vi "Receive.vi"(8 "error in (no error)":errorcluster, 10 "Transfer Group in":refnum<class "Transfer Group.lvclass">, 11 "PXImc Transceiver in":refnum<class "PXImc Transceiver.lvclass">) -> (0 "error out":errorcluster, 2 "Transfer Group out":refnum<class "Transfer Group.lvclass">, 3 "PXImc Transceiver out":refnum<class "PXImc Transceiver.lvclass">)   [LabVIEW 2017, in "PXImc.lvlib" / "PXImc Transceiver.lvclass"]
uses:
  PXImc Transceiver.lvclass
  Builds/Data Sharing Framework/Current/Core/DSF Core.lvlibp/Classes/Transfer Group/Transfer Group.lvclass
  PXImc Transceiver.lvclass/PXImc Transceiver.ctl
  <vilib>/pximc/Acquire Read Region (U8).vi
  <vilib>/pximc/nipximc.lvlib
  Builds/Data Sharing Framework/Current/Core/DSF Core.lvlibp/Classes/Buffer/Buffer.lvclass
  Builds/Data Sharing Framework/Current/Core/DSF Core.lvlibp/Classes/Transfer/Transfer.lvclass
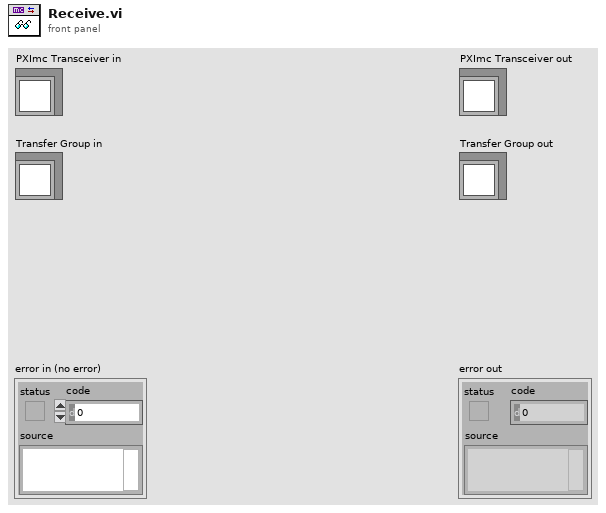
[diagram p1: front panel]
types:
  T1 = typedef "PXImc.lvlib/PXImc Transceiver.lvclass/PXImc Group Data.ctl" = cluster{"direction":T2, "transfers":T3[]}
  T2 = typedef "DSF Core.lvlibp/DSF Direction.ctl" = enum8{"Tx", "Rx"}
  T3 = typedef "PXImc.lvlib/PXImc Transceiver.lvclass/PXImc Transfer Data.ctl" = cluster{"stream id":u16, "session":refnum<k21>, "buffer size":u64}
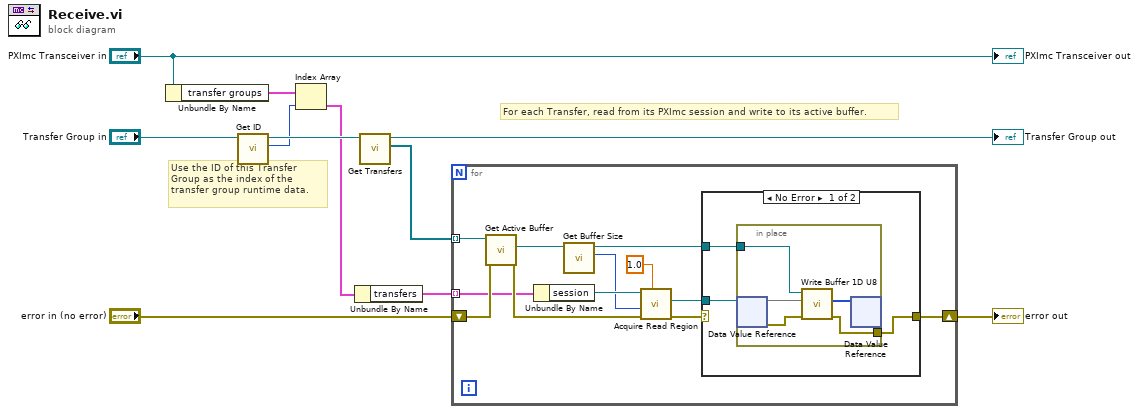
[diagram p0: block diagram]
diagram:
  # "For each Transfer, read from its PXImc session and write to its active buffer."
  # "Use the ID of this Transfer Group as the index of the transfer group runtime data."
  n1 = Unbundle By Name("PXImc Transceiver in") -> ("transfer groups"=w9:T1[])
  n2 = call "Get ID.vi"("Transfer Group in"="Transfer Group in") -> ("id"=w4:i32, "Transfer Group out"=w7:refnum<class "Transfer Group.lvclass">)  [unwired: 9 in]
  n3 = Index Array(array=w9, index=w4) -> (element=w3:T1)
  n4 = Unbundle By Name(w3) -> ("transfers"=w8:T3[])
  n5 = call "Get Transfers.vi"("Transfer Group in"=w7) -> ("Transfers"=w2:refnum<class "Transfer.lvclass">[], "Transfer Group out"=→"Transfer Group out":refnum<class "Transfer Group.lvclass">)  [unwired: 9 in]
  n6 = for {
    tunnel: w2 -> [w16] mode=indexing
    tunnel: w8 -> [w12] mode=indexing
    shift-right: [w19] -> w5
    shift-left: "error in (no error)" -> [w14]
    n7 = call "Get Active Buffer.vi"("error in (no error)"=w14, "Transfer in"=w16) -> ("error out"=w13:errorcluster, "Buffer"=w15:refnum<class "Buffer.lvclass">)  [unwired: 7 in, 1 out]
    n8 = Unbundle By Name(w12) -> ("session"=w23:refnum<k21>)
    n9 = call "Get Buffer Size.vi"("Buffer in"=w15) -> ("buffer size"=w21:u64, "Buffer out"=w17:refnum<class "Buffer.lvclass">)  [unwired: 9 in]
    n10 = call-poly <vilib>:"Acquire Read Region.vi"("timeout in seconds (5)"=1.0, "error in (no error)"=w13, "number of elements"=w21, "session in"=w23) -> ("error out"=w20:errorcluster, "read region reference"=w18:refnum<data-value>)  [unwired: 4 in, 2 out]
    n11 = case shown="No Error" w20 {
      selector: w20 -> [_ w32]
      tunnel: w18 -> [w26 _]
      tunnel: [w24 w32] -> w19
      tunnel: w17 -> [w25 _]
      frame No Error {
        n12 = in-place {
          in-place-border: w25 -> [w31]
          in-place-border: [w27] -> w24
          n13 = in-place-dvr #1(w26) -> (w29:u8[], w30:errorcluster)
          n14 = call "Write Buffer 1D U8.vi"("error in (no error)"=w30, "src array in"=w29, "Buffer in"=w31) -> ("error out"=w27:errorcluster, "src array out"=w28:u8[])  [unwired: 5 in, 2 out]
          n15 = in-place-dvr #1(w28) -> ()  [unwired: 2 out]
        }
      }
      frame Error {
      }
    }
  }
  "error out" <- w5
  "PXImc Transceiver out" <- "PXImc Transceiver in"
